vi "生成excel.vi"(1 "错误输入（无错误）":errorcluster, 2 "测试说明界面参数":T1) -> (0 "错误输出":errorcluster)   [LabVIEW 2015]
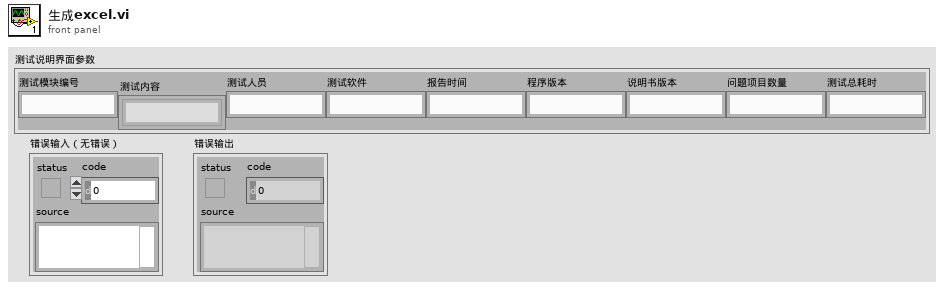
[diagram p1: front panel]
types:
  T1 = typedef "测试说明界面参数.ctl" = cluster{"测试模块编号":string, "测试内容":string[], "测试人员":string, "测试软件":string, "报告时间":string, "程序版本":string, "说明书版本":string, "问题项目数量":string, "测试总耗时":string}
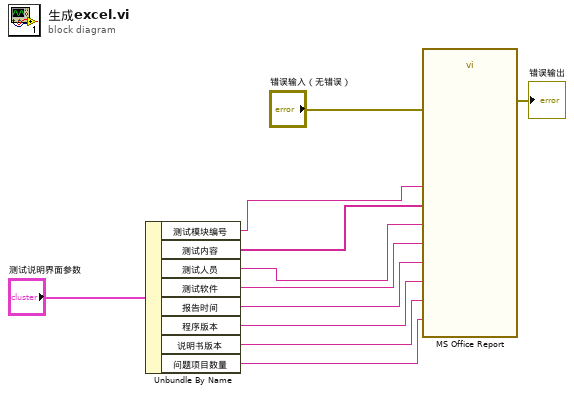
[diagram p0: block diagram]
diagram:
  n1 = Unbundle By Name("测试说明界面参数") -> ("测试模块编号"=w2:string, "测试内容"=w1:string[], "测试人员"=w8:string, "测试软件"=w7:string, "报告时间"=w6:string, "程序版本"=w5:string, "说明书版本"=w4:string, "问题项目数量"=w3:string)
  n2 = call "MS Office Report"("测试模块编号"=w2, "测试内容"=w1, "测试人员"=w8, "测试软件"=w7, "测试时间"=w6, "error in (no error)"="错误输入（无错误）", "程序版本"=w5, "说明书版本"=w4, "问题项目"=w3) -> ("error out"=→"错误输出":errorcluster)  [unwired: 18 in]
